vi "Initialize Attributes.vi"(8 "error in (no error)":errorcluster, 10 "Attribute Data":variant, 11 "LS218 in":refnum<class "LS218.lvclass">) -> (0 "error out":errorcluster, 2 "Found?":bool, 3 "LS218 out":refnum<class "LS218.lvclass">)   [LabVIEW 2015, in "LS218.lvlib" / "LS218.lvclass"]
doc: "Initialize object attribute.\n\nUnique resources should be allocated elsewhere!"
uses:
  LS218.lvclass
  PV-Enum.ctl
  CSPP_Core/Classes/CS++ProcessVariables/ProcessVariable/PV.lvclass
  CSPP_Core/Classes/CS++ProcessVariables/ProcessVariable/PV.lvclass/PV.ctl
  CSPP_Core/Actors/CS++BaseActor/CS++BaseActor.lvclass/CS++BaseActor.ctl
  LS218.lvclass/LS218.ctl
  CSPP_Core/Classes/CS++ProcessVariables/ProcessVariable/Write PV URL.vi
  CSPP_Core/Classes/CS++ProcessVariables/ProcessVariable/Write Type Descriptor.vi
  <vilib>/Utility/error.llb/Error Cluster From Error Code.vi
  CSPP_Core/Actors/CS++DeviceActor/CS++DeviceActor.lvclass
  CSPP_Core/Classes/CS++BaseClasses/Factory/CS++Factory.lvclass
  CSPP_Core/Classes/CS++ProcessVariables/CS++ProcessVariables.lvlib
  CSPP_Core/Actors/CS++BaseActor/CS++BaseActor.lvclass
panel:
  in  "PV-Enum":T1
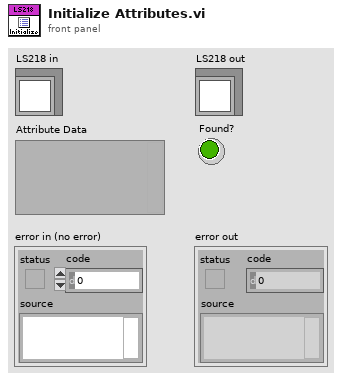
[diagram p1: front panel]
types:
  T1 = typedef "LS218.lvlib/LS218.lvclass/PV-Enum.ctl" = enum16{"T0", "T1", "T2", "T3", "T4", "T5", "T6", "T7", "Relay", "S0", "S1", "S2", "S3", "S4", "S5", "S6", "S7"}
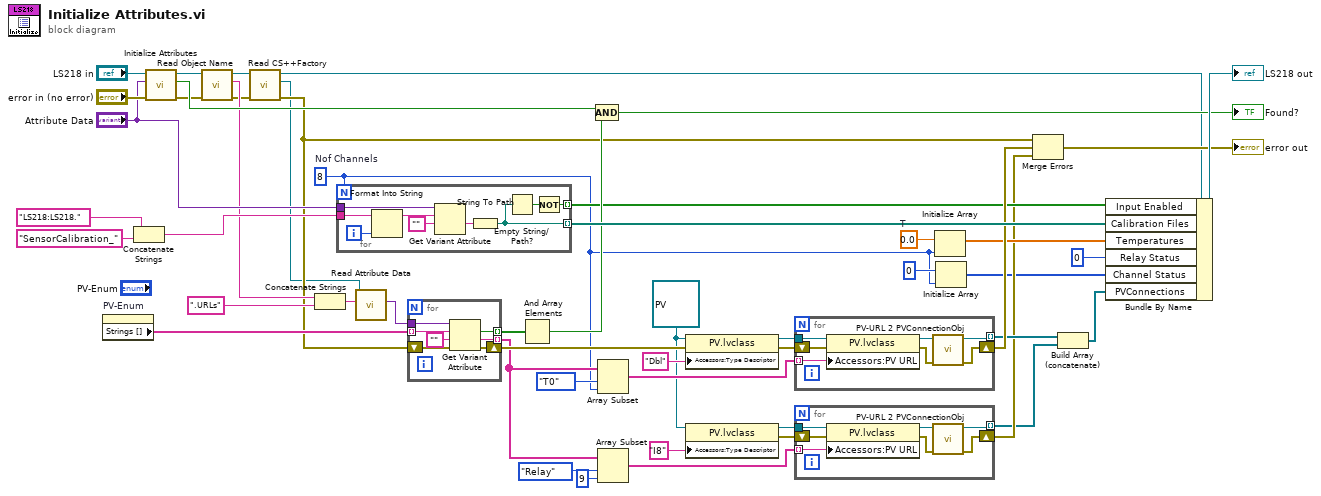
[diagram p0: block diagram]
diagram:
  w18 = dbl[unit] 0.0  # T
  w13 = refnum<class "PV.lvclass"> refnum ("CS++ProcessVariables.lvlib:PV.lvclass")
  w2 = 8  # Nof Channels
  n1 = property on="PV-Enum" class="Enum (strict)"() -> ("Strings []"=w30:string[])  [unwired: 2 in, 2 out]
  n2 = Concatenate Strings("LS218:LS218.", "SensorCalibration_" ("string")) -> (w46:string)
  n3 = call-parent "Initialize Attributes.vi"("error in (no error)"="error in (no error)", "Attribute Data"="Attribute Data", "CS++DeviceActor in"="LS218 in") -> ("error out"=w35:errorcluster, "Found?"=w51:bool, "CS++DeviceActor out"=w36:refnum<class "LS218.lvclass">)  [unwired: 6 in]
  n4 = call "Read Object Name.vi"("error in (no error)"=w35, "CS++BaseActor in"=w36) -> ("error out"=w21:errorcluster, "Object Name"=w31:string, "CS++BaseActor out"=w23:refnum<class "LS218.lvclass">)  [unwired: 7 in]
  n5 = call "Read CS++Factory.vi"("error in (no error)"=w21, "CS++BaseActor in"=w23) -> ("error out"=w20:errorcluster, "CS++Factory"=w19:refnum<class "CS++Factory.lvclass">, "CS++BaseActor out"=w22:refnum<class "LS218.lvclass">)  [unwired: 7 in]
  n6 = Concatenate Strings(w31, ".URLs" ("string")) -> (w38:string)
  n7 = for {
    N: w2 -> [_]
    tunnel: w46 -> [w60]
    tunnel: "Attribute Data" -> [w57]
    tunnel: [w54] -> w44 mode=indexing
    tunnel: [w52] -> w25 mode=indexing
    i -> [w59]
    n8 = Format Into String(initial string=w60, w59) -> (resulting string=w58:string)  [unwired: 2 in, 1 out]
    n9 = Get Variant Attribute(Variant=w57, name=w58, default value (empty Variant)="") -> (value=w55:string)  [unwired: 1 in, 3 out]
    n10 = String To Path(string=w55) -> (path=w54:path)
    n11 = Empty String/Path?(string/path=w54) -> (empty?=w53:bool)
    n12 = Not(x=w53) -> (.not. x?=w52:bool)
  }
  n13 = call-dynamic "Read Attribute Data.vi"("Object Name"=w38, "CS++Factory in"=w19) -> ("Attribute Data"=w29:variant)  [unwired: 7 in, 2 out]
  n14 = for {
    tunnel: [w66] -> w28 mode=indexing
    shift-right: [w67] -> w32
    shift-left: w20 -> [w65]
    tunnel: w30 -> [w63] mode=indexing
    tunnel: w29 -> [w64]
    tunnel: [w61] -> w10 mode=indexing
    n15 = Get Variant Attribute(Variant=w64, name=w63, default value (empty Variant)="", error in=w65) -> (found=w66:bool, value=w61:string, error out=w67:errorcluster)  [unwired: 1 out]
  }
  n16 = And Array Elements(Boolean array=w28) -> (logical AND=w33:bool)
  n17 = Compound Arithmetic op=AND(w51, w33) -> (→"Found?":bool)
  n18 = Array Subset(array=w10, index=PV-Enum."T0" ("PV-Enum"), length=w2) -> (w42:string[])
  n19 = Array Subset(array=w10, index=PV-Enum."Relay" ("PV-Enum"), length=9) -> (w11:string[])
  n20 = property class="PV.lvclass"(reference=w13, error in=w32, "Accessors:Type Descriptor"="Dbl" ("Type Descriptor")) -> (reference out=w40:refnum<class "PV.lvclass">, error out=w39:errorcluster)
  n21 = property class="PV.lvclass"(reference=w13, "Accessors:Type Descriptor"="I8" ("Type Descriptor")) -> (reference out=w15:refnum<class "PV.lvclass">, error out=w16:errorcluster)  [unwired: 1 in]
  n22 = for {
    tunnel: w40 -> [w74]
    tunnel: w42 -> [w73] mode=indexing
    tunnel: [w72] -> w24 mode=indexing
    shift-right: [w71] -> w26
    shift-left: w39 -> [w70]
    n23 = property class="PV.lvclass"(reference=w74, error in=w70, "Accessors:PV URL"=w73) -> (reference out=w69:refnum<class "PV.lvclass">, error out=w68:errorcluster)
    n24 = call "PV-URL 2 PVConnectionObj.vi"("Error In"=w68, "PV"=w69) -> ("Error Out"=w71:errorcluster, "PVConnection"=w72:refnum<class "PVConnection.lvclass">)  [unwired: 7 in, 1 out]
  }
  n25 = for {
    tunnel: w15 -> [w81]
    tunnel: w11 -> [w80] mode=indexing
    tunnel: [w79] -> w7 mode=indexing
    shift-right: [w78] -> w9
    shift-left: w16 -> [w77]
    n26 = property class="PV.lvclass"(reference=w81, error in=w77, "Accessors:PV URL"=w80) -> (reference out=w76:refnum<class "PV.lvclass">, error out=w75:errorcluster)
    n27 = call "PV-URL 2 PVConnectionObj.vi"("Error In"=w75, "PV"=w76) -> ("Error Out"=w78:errorcluster, "PVConnection"=w79:refnum<class "PVConnection.lvclass">)  [unwired: 7 in, 1 out]
  }
  n28 = Initialize Array(w18, w2) -> (w17:dbl[unit][])
  n29 = Initialize Array(i8 0, w2) -> (w1:i8[])
  n30 = Merge Errors(w20, w26, w9) -> (→"error out":errorcluster)
  n31 = Build Array (concatenate)(w24, w7) -> (w8:refnum<class "PVConnection.lvclass">[])
  n32 = Bundle By Name(cluster=w22, "Input Enabled"=w25, "Calibration Files"=w44, "Temperatures"=w17, "Relay Status"=u8 0, "Channel Status"=w1, "PVConnections"=w8) -> (→"LS218 out":refnum<class "LS218.lvclass">)
